vi "Set Serial Settings.vi"(8 "error IO":errorcluster, 10 "Serial Configuration":T1={"VISA"="", "Interface Type"=0, "Serial Interface"={"Baud Rate"=19200, "Data Bits "=8, "Parity"=enum."None", "Stop Bits"=0}, "Slave Address"=1} {"Interface Type" items=["GPIB"=1, "VXI"=2, "GPIB-VXI"=3, "Serial"=4, "PXI"=5, "TCPIP"=6, "USB"=7, "FireWire"=9, "Invalid"=0]; "Serial Interface"."Stop Bits" items=["1.0", "1.5", "2.0"]; "Serial Interface"."Baud Rate" items=["1200"=1200, "2400"=2400, "4800"=4800, "9600"=9600, "19200"=19200, "38400"=38400, "57600"=57600, "115200"=115200]; "Slave Address" format="%.0x"}, 11 "Module Configuration":refnum<class "Module Configuration.lvclass">) -> (0 "error IO out":errorcluster, 3 "Module Configuration out":refnum<class "Module Configuration.lvclass">)   [LabVIEW 2020, in "Plugin.lvlib" / "Plugin_UI.lvclass"]
doc: "Set Serial Settings"
uses:
  Plugin_UI.lvclass
  Serial Configuration.ctl
  builds/Libraries/Shared GUI Library.lvlibp/Shared GUI Library/Instrument Settings/Interface/Interface Type.ctl
  builds/Libraries/Shared GUI Library.lvlibp/Shared GUI Library/Instrument Settings/Interface/Serial Interafce.ctl
  builds/Libraries/LabSys Framework.lvlibp/Configuration Storage/Module Configuration/Module Configuration.lvclass
  builds/Libraries/Shared GUI Library.lvlibp
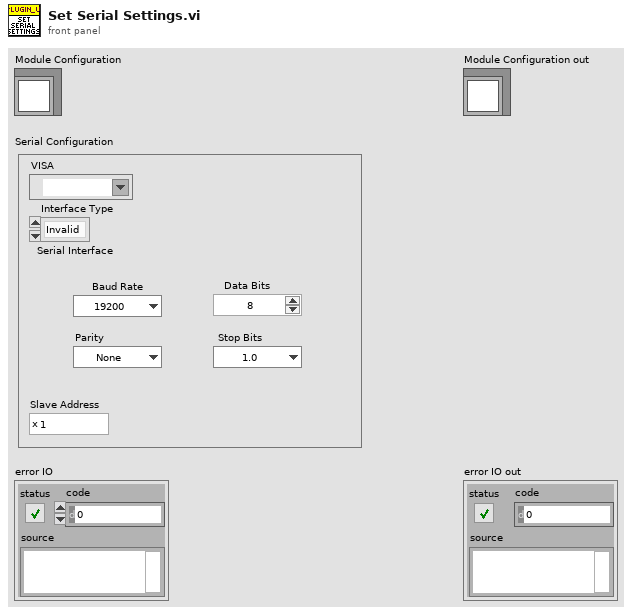
[diagram p1: front panel]
types:
  T1 = typedef "Plugin.lvlib/Plugin_UI.lvclass/Serial Configuration.ctl" = cluster{"VISA":refnum<visa-resource-name>, "Interface Type":T2, "Serial Interface":T3, "Slave Address":u8}
  T2 = typedef "Shared GUI Library.lvlibp/Interface Type.ctl" = u16
  T3 = typedef "Shared GUI Library.lvlibp/Serial Interafce.ctl" = cluster{"Baud Rate":u32, "Data Bits ":u16, "Parity":enum16{"None", "Odd", "Even"}, "Stop Bits":u16}
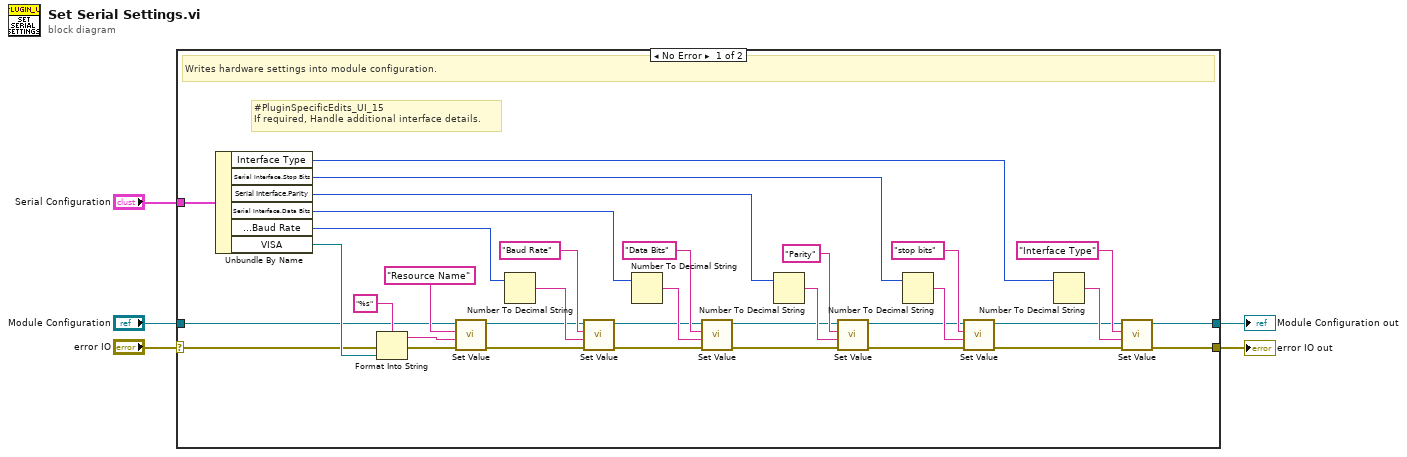
[diagram p0: block diagram]
diagram:
  n1 = case shown="No Error" "error IO" {
    selector: "error IO" -> [w10 w42]
    tunnel: [w6 w42] -> w1
    tunnel: "Module Configuration" -> [w9 w41]
    tunnel: [w7 w41] -> w2
    tunnel: "Serial Configuration" -> [w8 _]
    frame No Error {
      # "#PluginSpecificEdits_UI_15\nIf required, Handle additional interface details."
      # "Writes hardware settings into module configuration."
      n2 = Unbundle By Name(w8) -> ("Interface Type"=w11:T2, "Serial Interface.Stop Bits"=w16:u16, "Serial Interface.Parity"=w17:enum16{"None", "Odd", "Even"}, "Serial Interface.Data Bits"=w18:u16, "Serial Interface.Baud Rate"=w19:u32, "VISA"=w20:refnum<visa-resource-name>)
      n3 = Format Into String(format string="%s", error in=w10, w20) -> (resulting string=w24:string, error out=w21:errorcluster)  [unwired: 1 in]
      n4 = call "Set Value.vi"("error in (no error)"=w21, "Value"=w24, "Key"="Resource Name", "Module Configuration in"=w9) -> ("error out"=w25:errorcluster, "Module Configuration out"=w26:refnum<class "Module Configuration.lvclass">)  [unwired: 6 in]
      n5 = Number To Decimal String(number=w19) -> (decimal integer string=w40:string)  [unwired: 1 in]
      n6 = call "Set Value.vi"("error in (no error)"=w25, "Value"=w40, "Key"="Baud Rate", "Module Configuration in"=w26) -> ("error out"=w35:errorcluster, "Module Configuration out"=w28:refnum<class "Module Configuration.lvclass">)  [unwired: 6 in]
      n7 = Number To Decimal String(number=w18) -> (decimal integer string=w38:string)  [unwired: 1 in]
      n8 = call "Set Value.vi"("error in (no error)"=w35, "Value"=w38, "Key"="Data Bits", "Module Configuration in"=w28) -> ("error out"=w34:errorcluster, "Module Configuration out"=w29:refnum<class "Module Configuration.lvclass">)  [unwired: 6 in]
      n9 = Number To Decimal String(number=w17) -> (decimal integer string=w37:string)  [unwired: 1 in]
      n10 = call "Set Value.vi"("error in (no error)"=w34, "Value"=w37, "Key"="Parity", "Module Configuration in"=w29) -> ("error out"=w33:errorcluster, "Module Configuration out"=w30:refnum<class "Module Configuration.lvclass">)  [unwired: 6 in]
      n11 = Number To Decimal String(number=w16) -> (decimal integer string=w32:string)  [unwired: 1 in]
      n12 = call "Set Value.vi"("error in (no error)"=w33, "Value"=w32, "Key"="stop bits", "Module Configuration in"=w30) -> ("error out"=w12:errorcluster, "Module Configuration out"=w13:refnum<class "Module Configuration.lvclass">)  [unwired: 6 in]
      n13 = Number To Decimal String(number=w11) -> (decimal integer string=w14:string)  [unwired: 1 in]
      n14 = call "Set Value.vi"("error in (no error)"=w12, "Value"=w14, "Key"="Interface Type", "Module Configuration in"=w13) -> ("error out"=w6:errorcluster, "Module Configuration out"=w7:refnum<class "Module Configuration.lvclass">)  [unwired: 6 in]
    }
    frame Error {
    }
  }
  "Module Configuration out" <- w2
  "error IO out" <- w1
